vi "Mayus-Minus.vi"() -> ()   [LabVIEW 2019]
uses:
  <vilib>/event_ctls.llb/eventvkey.ctl
panel:
  out "*(type *) &x":string
  out "VKey":T1
  out "Letras":string
  in  "Teclas":string
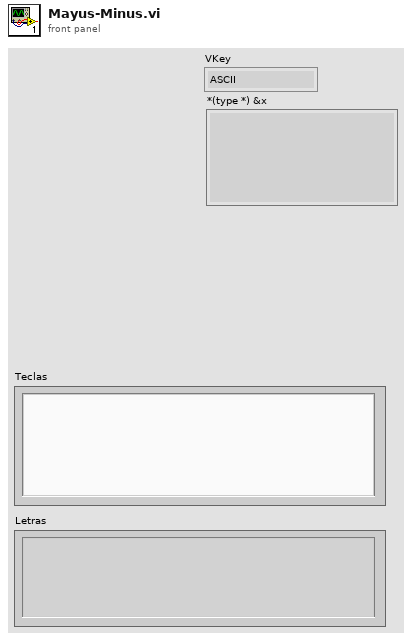
[diagram p1: front panel]
types:
  T1 = typedef "eventvkey.ctl" = enum16{"ASCII", "Enter", "Return", "Shift", "Ctrl", "Alt", "Cmd", "Opt", "Caps", "NumLock", "Clear", "Break", "Up", "Down", "Left", "Right", "Insert", "Delete", "Home", "End", "PageUp", "PageDown", "Escape", "Help", "Pause", "ScrollLock", "F1", "F2", "F3", "F4", "F5", "F6", "F7", "F8", "F9", "F10", "F11", "F12", "F13", "F14", "F15", "F16", "F17", "F18", "F19", "F20", "F21", "F22", "F23", "F24", "Play", "VolumeUp", "VolumeDown", "Mute", "Two Byte Char"}
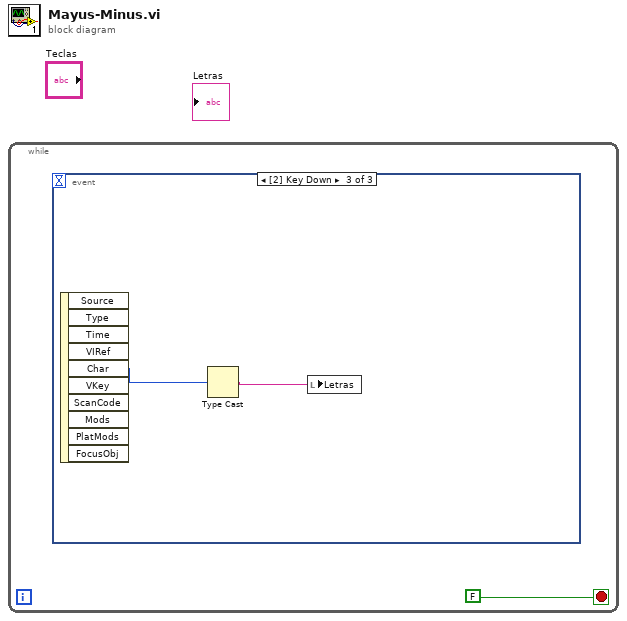
[diagram p0: block diagram]
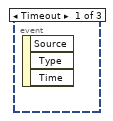
[diagram p2: hidden frame]
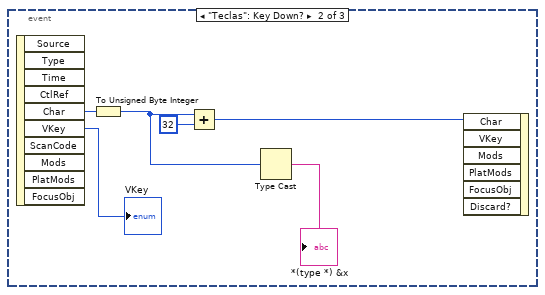
[diagram p3: hidden frame]
diagram:
  n1 = while {
    stop <- FALSE stop-if-true
    n2 = event shown="[2] Key Down" {
      selector: _ -> [_ _ _]
      dyn-events: _ -> [_ _ _]
      timeout: _ -> [_ _ _]
      event Timeout {
        n3 = event-data() -> ()  [unwired: 1 in, 3 out]
      }
      event "Teclas": Key Down? {
        n4 = event-data() -> ("Char"=w6:i16, "VKey"=→"VKey":T1)  [unwired: 1 in, 8 out]
        n5 = To Unsigned Byte Integer(number=w6) -> (unsigned 8bit integer=w3:u8)
        n6 = Add(x=w3, y=u8 32) -> (x+y=w4:u8)
        n7 = Type Cast(x=w3) -> (*(type *) &x=→"*(type *) &x":string)  [unwired: 1 in]
        n8 = event-data("Char"=w4) -> ()  [unwired: 6 in, 1 out]
      }
      event Key Down {
        n9 = event-data() -> ("Char"=w8:i16)  [unwired: 1 in, 9 out]
        n10 = Type Cast(x=w8) -> (*(type *) &x=w9:string)  [unwired: 1 in]
        n11 = local write "Letras"(w9) -> ()
      }
    }
  }
